vi "Swerve Drive Main.vi"(0 "Drive Joystick":string="My Joystick RefNum") -> ()   [LabVIEW 2018]
uses:
  Angle offsets.ctl
  <vilib>/Rock Robotics/WPI/Utilities/WPI_GetSetVariantRefNum.vi
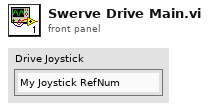
[diagram p1: front panel]
types:
  T1 = typedef "Angle offsets.ctl" = cluster{"FR Offset":dbl, "FL Offset":dbl, "RL Offset":dbl, "RR Offset":dbl}
  T2 = typedef "WPI_JoystickDevRef.ctl" = cluster{"Device":T3}
  T3 = typedef "WPI_JoystickDeviceEnum.ctl" = enum16{"USB 0", "USB 1", "USB 2", "USB 3", "USB 4", "USB 5"}
  T4 = typedef "Encoder Unpacked Data.ctl" = cluster{"FR ENC":dbl, "FL ENC":dbl, "RL ENC":dbl, "RR ENC":dbl}
  T5 = typedef "Motor Data Unpacked.ctl" = cluster{"FR DP":dbl, "FR ANG":dbl, "FL DP":dbl, "FL ANG":dbl, "RL DP":dbl, "RL ANG":dbl, "RR DP":dbl, "RR ANG":dbl}
  T6 = typedef "Final Motor Data.ctl" = cluster{"Drive Power":dbl, "Goal Angle":dbl, "Real Angle":dbl}
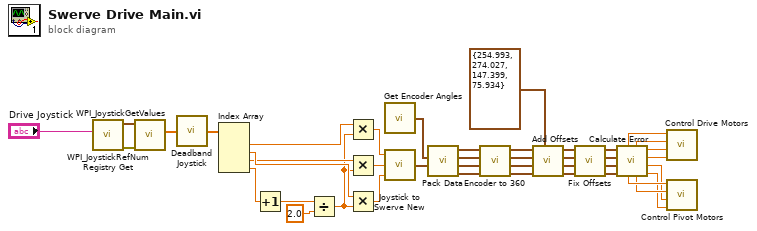
[diagram p0: block diagram]
diagram:
  n1 = call <vilib>:"WPI_JoystickRefNum Registry Get.vi"("refnum name"="Drive Joystick") -> ("error out"=w41:errorcluster, "JoystickDevRef"=w40:T2)  [unwired: 9 in]
  n2 = call <vilib>:"WPI_JoystickGetValues.vi"("error in (no error)"=w41, "JoystickDevRef"=w40) -> ("Axes"=w13:dbl[])  [unwired: 5 in, 4 out]
  n3 = call "Deadband Joystick.vi"("Axes"=w13) -> ("Axes"=w12:dbl[])
  n4 = Index Array(array=w12) -> (element #1=w8:dbl, element #2=w7:dbl, element #3=w6:dbl, element #4=w11:dbl)  [unwired: 4 in]
  n5 = Increment(x=w11) -> (x+1=w10:dbl)
  n6 = Divide(x=w10, y=2.0) -> (x/y=w5:dbl)
  n7 = Multiply(x=w8, y=w5) -> (x*y=w4:dbl)
  n8 = Multiply(x=w6, y=w5) -> (x*y=w2:dbl)
  n9 = Multiply(x=w7, y=w5) -> (x*y=w3:dbl)
  n10 = call "Get Encoder Angles.vi"() -> ("output cluster"=w39:T4)
  n11 = call "Joystick to Swerve New.vi"("Joystick Y"=w3, "Joystick R"=w2, "Joystick X"=w4) -> ("output cluster"=w1:T5)
  n12 = call "Pack Data.vi"("Math"=w1, "Encoder"=w39) -> ("RR Data"=w34:T6, "RL Data"=w35:T6, "FL Data"=w36:T6, "FR Data"=w37:T6)  [unwired: 2 in]
  n13 = call "Encoder to 360.vi"("Rear Right Data"=w34, "Rear Left Data"=w35, "Front Left Data"=w36, "Front Right Data"=w37) -> ("Rear Right Data"=w33:T6, "Rear Left Data"=w32:T6, "Front Left Data"=w31:T6, "Front Right Data"=w30:T6)
  n14 = call "Add Offsets.vi"("Cluster"=T1 {"FR Offset"=254.993, "FL Offset"=274.027, "RL Offset"=147.399, "RR Offset"=75.934}, "RR Data"=w33, "RL Data"=w32, "FL Data"=w31, "FR Data"=w30) -> ("RR Data Out"=w26:T6, "RL Data Out"=w27:T6, "FL Data Out"=w28:T6, "FR Data Out"=w29:T6)
  n15 = call "Fix Offsets.vi"("Rear Right"=w26, "Rear Left"=w27, "Front Left"=w28, "Front Right"=w29) -> ("Rear Right"=w22:T6, "Rear Left"=w23:T6, "Front Left"=w24:T6, "Front Right"=w25:T6)
  n16 = call "Calculate Error.vi"("Rear Right"=w22, "Rear Left"=w23, "Front Left"=w24, "Front Right"=w25) -> ("Rear Right Angle Error"=w14:dbl, "Rear Left Angle Error"=w15:dbl, "Rear Right Drive Power"=w18:dbl, "Rear Left Drive Power"=w19:dbl, "Front Left Angle Error"=w16:dbl, "Front Left Drive Power"=w20:dbl, "Front Right Angle Error"=w17:dbl, "Front Right Drive Power"=w21:dbl)
  n17 = call "Control Drive Motors.vi"("Rear Right Power"=w18, "Rear Left Power"=w19, "Front Left Power"=w20, "Front Right Power"=w21) -> ()
  n18 = call "Control Pivot Motors.vi"("Rear Right Error"=w14, "Rear Left Error"=w15, "Front Left Error"=w16, "Front Right Error"=w17) -> ()
